vi "Set Item Property (Dependent File).vi"(6 "OptionalInfo":T1, 8 "error in (no error)":errorcluster, 9 "Path":path, 10 "Property Name":string, 11 "Item Ref in":T2 format="%.0x") -> (0 "error out":errorcluster, 3 "Item Ref out":T2 format="%.0x", 4 "Replaced":bool)   [LabVIEW 2020, in "Custom Device API.lvlib"]
doc: "Sets a <B>Property Name</B> and <B>Value</B> for an item property and saves this information in the system definition file. If the <B>Property Name</B> you specify already exists, this VI overwrites the property. Wire data to the <B>Value</B> input to determine the polymorphic instance to use or manually select the instance."
uses:
  <vilib>/NI VeriStand/Custom Device API/Custom Device API.lvlib
  <vilib>/NI VeriStand/Custom Device API/Custom Device Item Ref.ctl
  <vilib>/NI VeriStand/Custom Device API/Dependent File Optional Info.ctl
  3ddfc329-f0c5-496b-bea5-9c44d07b9d50.vi
  <vilib>/NI VeriStand/Custom Device API/Custom Device Offline Path.vi
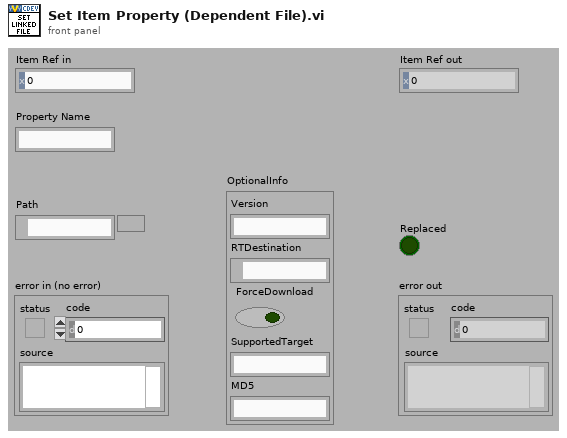
[diagram p1: front panel]
types:
  T1 = typedef "Custom Device API.lvlib/Dependent File Optional Info.ctl" = cluster{"Version":string, "RTDestination":path, "ForceDownload":bool, "SupportedTarget":string, "MD5":string}
  T2 = typedef "Custom Device API.lvlib/Custom Device Item Ref.ctl" = u64
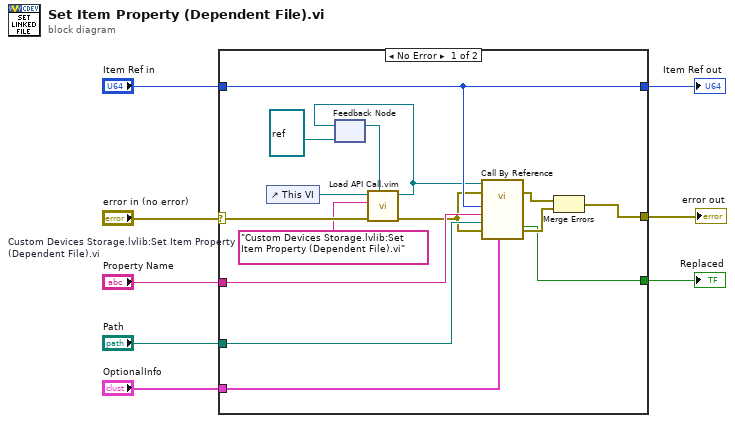
[diagram p0: block diagram]
diagram:
  n1 = case shown="No Error" "error in (no error)" {
    selector: "error in (no error)" -> [w14 w25]
    tunnel: "Item Ref in" -> [w17 w24]
    tunnel: [w17 w24] -> w7
    tunnel: [w22 w25] -> w6
    tunnel: "Property Name" -> [w21 _]
    tunnel: "Path" -> [w20 _]
    tunnel: [w19 _] -> w3
    tunnel: "OptionalInfo" -> [w18 _]
    frame No Error {
      w10 = "Custom Devices Storage.lvlib:Set Item Property (Dependent File).vi"  # Custom Devices Storage.lvlib:Set Item Property (Dependent File).vi
      n2 = control-ref of="This VI"() -> (w15:refnum<vi>)
      n3 = feedback #1(refnum<vi> refnum ("type specifier VI Refnum (for type only)")) -> (w16:refnum<vi>)
      n4 = call "Load API Call.vim"("VI reference in"=w16, "error in (no error)"=w14, "VI qualified name"=w10, "Caller VI ref"=w15) -> ("error out"=w13:errorcluster, "VI reference"=w12:refnum<vi>)  [unwired: 6 in]
      n5 = feedback-in #1(w12) -> ()
      n6 = call-by-ref "?"(reference=w12, error in=w13, "OptionalInfo"=w18, 8:"error in (no error)"=w13, "Path"=w20, "Property Name"=w21, "Item Ref in"=w17) -> (error out=w9:errorcluster, 0:"error out"=w23:errorcluster, "Replaced"=w19:bool)  [unwired: 4 in, 2 out]
      n7 = Merge Errors(w9, w23) -> (w22:errorcluster)
    }
    frame Error {
    }
  }
  "Item Ref out" <- w7
  "error out" <- w6
  "Replaced" <- w3
